vi "colour.vi"(7 "Colour":T2(ring), 8 "error in":errorcluster, 9 "Range":cluster{u32, u32}(slide)={65535, 0} scale=0.0..65535.0, 10 "image":u16[][](array[numeric])) -> (0 "error thru":errorcluster, 2 "picture":picture, 5 "stats":T1={"Histogram"={"X Values"=[5479.58, 5926.74, 6373.9, 6821.06, 7268.22, 7715.38, 8162.54, 8609.7, 9056.86, 9504.02, 9951.18, 10398.34, 10845.5, 11292.66, 11739.82, 12186.98, 12634.14, 13081.3, 13528.46, 13975.62, 14422.78, 14869.94, 15317.1, 15764.26, 16211.42, 16658.58, 17105.74, 17552.9, 18000.06, 18447.22, 18894.38, 19341.54, 19788.7, 20235.86, 20683.02, 21130.18, 21577.34, 22024.5, 22471.66, 22918.82, 23365.98, 23813.14, 24260.3, 24707.46, 25154.62, 25601.78, 26048.94, 26496.1, 26943.26, 27390.42, 27837.58, 28284.74, 28731.9, 29179.06, 29626.22, 30073.38, 30520.54, 30967.7, 31414.86, 31862.02, 32309.18, 32756.34, 33203.5, 33650.66, 34097.82, 34544.98, 34992.14, 35439.3, 35886.46, 36333.62, 36780.78, 37227.94, 37675.1, 38122.26, 38569.42, 39016.58, 39463.74, 39910.9, 40358.06, 40805.22, 41252.38, 41699.54, 42146.7, 42593.86, 43041.02, 43488.18, 43935.34, 44382.5, 44829.66, 45276.82, 45723.98, 46171.14, 46618.3, 47065.46, 47512.62, 47959.78, 48406.94, 48854.1, 49301.26, 49748.42], "Histogram: h(x)"=[2, 4, 12, 22, 46, 28, 40, 61, 53, 89, 50, 76, 48, 43, 66, 54, 64, 43, 68, 121, 142, 240, 196, 324, 218, 283, 392, 283, 484, 412, 686, 750, 950, 1540, 1320, 2011, 1718, 1854, 2735, 2129, 3147, 3035, 5720, 5312, 5580, 7214, 5907, 10090, 10110, 12384, 18538, 16232, 29146, 28690, 37550, 21004, 14573, 14196, 8331, 8677, 4932, 5351, 3336, 2737, 2709, 1284, 1035, 366, 207, 109, 29, 9, 1, 0, 0, 0, 0, 0, 0, 0, 0, 0, 0, 0, 0, 0, 0, 0, 0, 0, 0, 0, 0, 0, 0, 0, 0, 0, 0, 1]}, "max value"=0, "min value"=0})   [LabVIEW 2020]
uses:
  _controls/stats.ctl
  _controls/cluster.range.sgl.ctl
  <vilib>/Analysis/NI_AALBase.lvlib
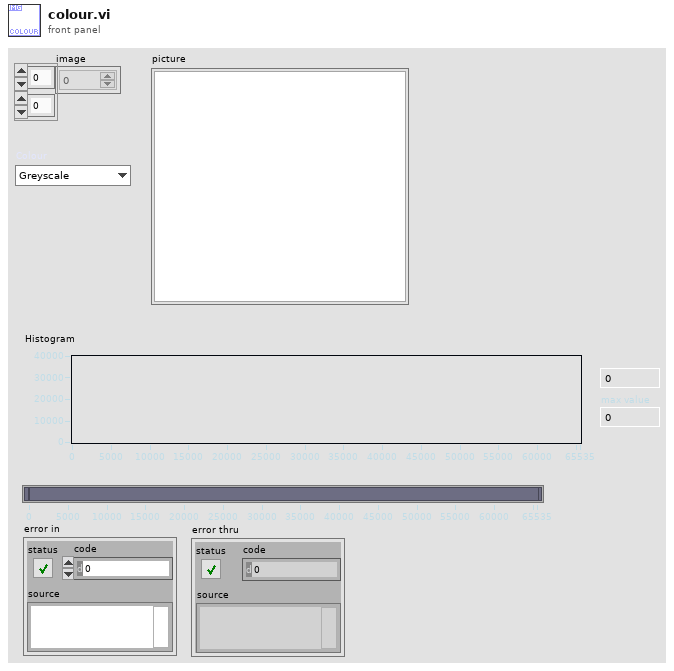
[diagram p1: front panel]
types:
  T1 = typedef "stats.ctl" = cluster{"Histogram":cluster{"X Values":dbl[], "Histogram: h(x)":i32[]}, "max value":u16, "min value":u16}
  T2 = enum16{"Greyscale", "Earth", "Fire", "Rainbow Inverted", "Rainbow", "Red Hot", "Water", "-", "Red", "Orange", "Yellow", "Green", "Cyan", "Blue", "Purple", "Pink"}
  T3 = typedef "cluster.range.sgl.ctl" = cluster{"min":sgl, "max":sgl}
  T4 = cluster{"X Values":dbl[], "Histogram: h(x)":i32[]}
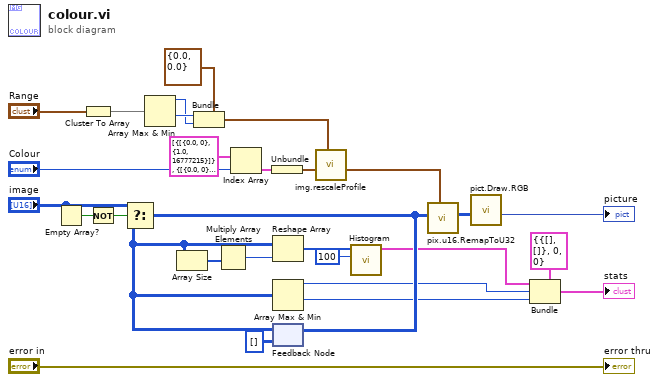
[diagram p0: block diagram]
diagram:
  n1 = Empty Array?(array="image") -> (empty?=w21:bool)
  n2 = Cluster To Array(cluster="Range") -> (array=w1:u32[])
  n3 = Not(x=w21) -> (.not. x?=w20:bool)
  n4 = Array Max & Min(array=w1) -> (max value=w3:u32, min value=w4:u32)  [unwired: 2 out]
  n5 = Bundle(cluster=T3 {"min"=0.0, "max"=0.0} ("range"), "min"=w4, "max"=w3) -> (w2:T3)
  n6 = Index Array(array=cluster{"MarkerValues":cluster{dbl, u32}[]}[] [{"MarkerValues"=[{0.0, 0}, {1.0, 16777215}]}, {"MarkerValues"=[{0.0, 0}, {1.0, 7}, {2.0, 15}, {3.0, 22}, {4.0, 30}, {5.0, 38}, {6.0, 45}, {7.0, 53}, {8.0, 61}, {9.0, 65}, {10.0, 69}, {11.0, 74}, {12.0, 78}, {13.0, 82}, {14.0, 87}, {15.0, 91}, {16.0, 65632}, {17.0, 262244}, {18.0, 458856}, {19.0, 655468}, {20.0, 852081}, {21.0, 1048693}, {22.0, 1245305}, {23.0, 1441917}, {24.0, 1638530}, {25.0, 1835142}, {26.0, 2031754}, {27.0, 2228367}, {28.0, 2424979}, {29.0, 2621591}, {30.0, 2818204}, {31.0, 3014816}, {32.0, 3211429}, {33.0, 3408040}, {34.0, 3604651}, {35.0, 3801263}, {36.0, 3997874}, {37.0, 4194485}, {38.0, 4391097}, {39.0, 4587708}, {40.0, 4784320}, {41.0, 4980931}, {42.0, 5177543}, {43.0, 5374154}, {44.0, 5570766}, {45.0, 5767377}, {46.0, 5963989}, {47.0, 6160600}, {48.0, 6422748}, {49.0, 6619356}, {50.0, 6815965}, {51.0, 7012574}, {52.0, 7209183}, {53.0, 7405792}, {54.0, 7602401}, {55.0, 7799010}, {56.0, 7995619}, {57.0, 8192224}, {58.0, 8388830}, {59.0, 8585436}, {60.0, 8782042}, {61.0, 8978648}, {62.0, 9175254}, {63.0, 9371860}, {64.0, 9568466}, {65.0, 9699534}, {66.0, 9830602}, {67.0, 9961671}, {68.0, 10092739}, {69.0, 10223807}, {70.0, 10354876}, {71.0, 10485944}, {72.0, 10617013}, {73.0, 10682545}, {74.0, 10748077}, {75.0, 10879145}, {76.0, 10944678}, {77.0, 11010210}, {78.0, 11141278}, {79.0, 11206810}, {80.0, 11337879}, {81.0, 11403411}, {82.0, 11468943}, {83.0, 11600012}, {84.0, 11665544}, {85.0, 11731076}, {86.0, 11862145}, {87.0, 11927677}, {88.0, 12058746}, {89.0, 12124278}, {90.0, 12189810}, {91.0, 12320879}, {92.0, 12386411}, {93.0, 12451943}, {94.0, 12583012}, {95.0, 12648544}, {96.0, 12779613}, {97.0, 12845401}, {98.0, 12976981}, {99.0, 13043026}, {100.0, 13174606}, {101.0, 13240394}, {102.0, 13371975}, {103.0, 13438019}, {104.0, 13569600}, {105.0, 13635644}, {106.0, 13701944}, {107.0, 13767989}, {108.0, 13899825}, {109.0, 13966125}, {110.0, 14032170}, {111.0, 14098470}, {112.0, 14230307}, {113.0, 14296351}, {114.0, 14428187}, {115.0, 14494487}, {116.0, 14626324}, {117.0, 14692368}, {118.0, 14824204}, {119.0, 14890504}, {120.0, 15022341}, {121.0, 15088388}, {122.0, 15154691}, {123.0, 15286531}, {124.0, 15352834}, {125.0, 15418881}, {126.0, 15550721}, {127.0, 15617024}, {128.0, 15748864}, {129.0, 15814912}, {130.0, 15946752}, {131.0, 16013056}, {132.0, 16144896}, {133.0, 16210944}, {134.0, 16342784}, {135.0, 16409088}, {136.0, 16540928}, {137.0, 16541440}, {138.0, 16541952}, {139.0, 16608000}, {140.0, 16608512}, {141.0, 16609024}, {142.0, 16675072}, {143.0, 16675584}, {144.0, 16741632}, {145.0, 16742144}, {146.0, 16742656}, {147.0, 16743168}, {148.0, 16743680}, {149.0, 16744192}, {150.0, 16744704}, {151.0, 16745216}, {152.0, 16745728}, {153.0, 16745984}, {154.0, 16746496}, {155.0, 16747008}, {156.0, 16747520}, {157.0, 16747776}, {158.0, 16748288}, {159.0, 16748800}, {160.0, 16749312}, {161.0, 16749568}, {162.0, 16750080}, {163.0, 16750592}, {164.0, 16751104}, {165.0, 16751360}, {166.0, 16751872}, {167.0, 16752384}, {168.0, 16752896}, {169.0, 16753152}, {170.0, 16753664}, {171.0, 16754176}, {172.0, 16754688}, {173.0, 16754944}, {174.0, 16755456}, {175.0, 16755968}, {176.0, 16756480}, {177.0, 16756736}, {178.0, 16757248}, {179.0, 16757760}, {180.0, 16758272}, {181.0, 16758784}, {182.0, 16759296}, {183.0, 16759808}, {184.0, 16760320}, {185.0, 16760576}, {186.0, 16761088}, {187.0, 16761600}, {188.0, 16762112}, {189.0, 16762624}, {190.0, 16763136}, {191.0, 16763648}, {192.0, 16764160}, {193.0, 16764416}, {194.0, 16764928}, {195.0, 16765440}, {196.0, 16765952}, {197.0, 16766208}, {198.0, 16766720}, {199.0, 16767232}, {200.0, 16767744}, {201.0, 16768000}, {202.0, 16768512}, {203.0, 16769024}, {204.0, 16769536}, {205.0, 16770048}, {206.0, 16770560}, {207.0, 16771072}, {208.0, 16771584}, {209.0, 16771844}, {210.0, 16772360}, {211.0, 16772877}, {212.0, 16773393}, {213.0, 16773653}, {214.0, 16774170}, {215.0, 16774686}, {216.0, 16775203}, {217.0, 16775210}, {218.0, 16775474}, {219.0, 16775738}, {220.0, 16776002}, {221.0, 16776266}, {222.0, 16776530}, {223.0, 16776794}, {224.0, 16777058}, {225.0, 16777065}, {226.0, 16777073}, {227.0, 16777081}, {228.0, 16777089}, {229.0, 16777096}, {230.0, 16777104}, {231.0, 16777112}, {232.0, 16777120}, {233.0, 16777127}, {234.0, 16777135}, {235.0, 16777143}, {236.0, 16777151}, {237.0, 16777159}, {238.0, 16777167}, {239.0, 16777175}, {240.0, 16777183}, {241.0, 16777187}, {242.0, 16777191}, {243.0, 16777195}, {244.0, 16777199}, {245.0, 16777203}, {246.0, 16777207}, {247.0, 16777211}, {248.0, 16777215}, {249.0, 16777215}, {250.0, 16777215}, {251.0, 16777215}, {252.0, 16777215}, {253.0, 16777215}, {254.0, 16777215}, {255.0, 16777215}]}, {"MarkerValues"=[{0.0, 0}, {21845.0, 16744277}, {43690.0, 16777130}, {65535.0, 16777215}]}, {"MarkerValues"=[{6.0, 63}, {5.0, 255}, {4.0, 65535}, {3.0, 65280}, {2.0, 16776960}, {1.0, 16711680}, {0.0, 8323072}]}, {"MarkerValues"=[{0.0, 0}, {1.0, 255}, {2.0, 65535}, {3.0, 65280}, {4.0, 16776960}, {5.0, 16711680}, {6.0, 8323072}]}, {"MarkerValues"=[{0.0, 0}, {1.0, 0}, {2.0, 0}, {3.0, 0}, {4.0, 65793}, {5.0, 65793}, {6.0, 65793}, {7.0, 65793}, {8.0, 65793}, {9.0, 262144}, {10.0, 458752}, {11.0, 655360}, {12.0, 851968}, {13.0, 1048576}, {14.0, 1310720}, {15.0, 1507328}, {16.0, 1769472}, {17.0, 1966080}, {18.0, 2162688}, {19.0, 2359296}, {20.0, 2555904}, {21.0, 2752512}, {22.0, 2949120}, {23.0, 3145728}, {24.0, 3407872}, {25.0, 3604480}, {26.0, 3801088}, {27.0, 3997696}, {28.0, 4259840}, {29.0, 4456448}, {30.0, 4653056}, {31.0, 4849664}, {32.0, 5111808}, {33.0, 5308416}, {34.0, 5505024}, {35.0, 5701632}, {36.0, 5898240}, {37.0, 6094848}, {38.0, 6291456}, {39.0, 6488064}, {40.0, 6750208}, {41.0, 6946816}, {42.0, 7208960}, {43.0, 7405568}, {44.0, 7667712}, {45.0, 7864320}, {46.0, 8060928}, {47.0, 8257536}, {48.0, 8519680}, {49.0, 8716288}, {50.0, 8912896}, {51.0, 9109504}, {52.0, 9306112}, {53.0, 9502720}, {54.0, 9699328}, {55.0, 9895936}, {56.0, 10158080}, {57.0, 10354688}, {58.0, 10551296}, {59.0, 10747904}, {60.0, 11010048}, {61.0, 11206656}, {62.0, 11403264}, {63.0, 11599872}, {64.0, 11862016}, {65.0, 12058624}, {66.0, 12255232}, {67.0, 12451840}, {68.0, 12648448}, {69.0, 12845056}, {70.0, 13107200}, {71.0, 13303808}, {72.0, 13565952}, {73.0, 13762560}, {74.0, 13959168}, {75.0, 14155776}, {76.0, 14417920}, {77.0, 14614528}, {78.0, 14811136}, {79.0, 15007744}, {80.0, 15269888}, {81.0, 15466496}, {82.0, 15663104}, {83.0, 15859712}, {84.0, 16056320}, {85.0, 16187392}, {86.0, 16384256}, {87.0, 16515584}, {88.0, 16712448}, {89.0, 16713216}, {90.0, 16713984}, {91.0, 16714752}, {92.0, 16715776}, {93.0, 16716544}, {94.0, 16717312}, {95.0, 16718080}, {96.0, 16719104}, {97.0, 16719872}, {98.0, 16720640}, {99.0, 16721408}, {100.0, 16722432}, {101.0, 16723200}, {102.0, 16723968}, {103.0, 16724736}, {104.0, 16725760}, {105.0, 16726528}, {106.0, 16727296}, {107.0, 16728064}, {108.0, 16729088}, {109.0, 16729856}, {110.0, 16730624}, {111.0, 16731392}, {112.0, 16732416}, {113.0, 16733184}, {114.0, 16733952}, {115.0, 16734720}, {116.0, 16735744}, {117.0, 16736512}, {118.0, 16737280}, {119.0, 16738048}, {120.0, 16738816}, {121.0, 16739584}, {122.0, 16740352}, {123.0, 16741120}, {124.0, 16742144}, {125.0, 16742912}, {126.0, 16743936}, {127.0, 16744704}, {128.0, 16745728}, {129.0, 16746496}, {130.0, 16747264}, {131.0, 16748032}, {132.0, 16748800}, {133.0, 16749568}, {134.0, 16750336}, {135.0, 16751104}, {136.0, 16752128}, {137.0, 16752896}, {138.0, 16753664}, {139.0, 16754432}, {140.0, 16755456}, {141.0, 16756224}, {142.0, 16756992}, {143.0, 16757760}, {144.0, 16758784}, {145.0, 16759552}, {146.0, 16760320}, {147.0, 16761088}, {148.0, 16762112}, {149.0, 16762880}, {150.0, 16763648}, {151.0, 16764416}, {152.0, 16765184}, {153.0, 16765952}, {154.0, 16766976}, {155.0, 16767744}, {156.0, 16768768}, {157.0, 16769536}, {158.0, 16770304}, {159.0, 16771072}, {160.0, 16772096}, {161.0, 16772864}, {162.0, 16773632}, {163.0, 16774400}, {164.0, 16775424}, {165.0, 16775681}, {166.0, 16776195}, {167.0, 16776452}, {168.0, 16776966}, {169.0, 16776969}, {170.0, 16776972}, {171.0, 16776975}, {172.0, 16776979}, {173.0, 16776982}, {174.0, 16776985}, {175.0, 16776988}, {176.0, 16776992}, {177.0, 16776995}, {178.0, 16776998}, {179.0, 16777001}, {180.0, 16777005}, {181.0, 16777008}, {182.0, 16777011}, {183.0, 16777014}, {184.0, 16777018}, {185.0, 16777021}, {186.0, 16777024}, {187.0, 16777027}, {188.0, 16777031}, {189.0, 16777034}, {190.0, 16777037}, {191.0, 16777040}, {192.0, 16777044}, {193.0, 16777047}, {194.0, 16777050}, {195.0, 16777053}, {196.0, 16777057}, {197.0, 16777060}, {198.0, 16777063}, {199.0, 16777066}, {200.0, 16777070}, {201.0, 16777073}, {202.0, 16777076}, {203.0, 16777079}, {204.0, 16777082}, {205.0, 16777085}, {206.0, 16777088}, {207.0, 16777091}, {208.0, 16777095}, {209.0, 16777098}, {210.0, 16777102}, {211.0, 16777105}, {212.0, 16777109}, {213.0, 16777112}, {214.0, 16777115}, {215.0, 16777118}, {216.0, 16777121}, {217.0, 16777124}, {218.0, 16777127}, {219.0, 16777130}, {220.0, 16777134}, {221.0, 16777137}, {222.0, 16777140}, {223.0, 16777143}, {224.0, 16777147}, {225.0, 16777150}, {226.0, 16777153}, {227.0, 16777156}, {228.0, 16777160}, {229.0, 16777163}, {230.0, 16777166}, {231.0, 16777169}, {232.0, 16777173}, {233.0, 16777176}, {234.0, 16777179}, {235.0, 16777182}, {236.0, 16777185}, {237.0, 16777188}, {238.0, 16777192}, {239.0, 16777195}, {240.0, 16777199}, {241.0, 16777202}, {242.0, 16777205}, {243.0, 16777208}, {244.0, 16777212}, {245.0, 16777212}, {246.0, 16777213}, {247.0, 16777214}, {248.0, 16777215}, {249.0, 16777215}, {250.0, 16777215}, {251.0, 16777215}, {252.0, 16777215}, {253.0, 16777215}, {254.0, 16777215}, {255.0, 16777215}]}, {"MarkerValues"=[{0.0, 0}, {1.0, 255}, {2.0, 16777215}]}, {"MarkerValues"=[]}, {"MarkerValues"=[{0.0, 0}, {1.0, 16711680}]}, {"MarkerValues"=[{0.0, 0}, {1.0, 16744448}]}, {"MarkerValues"=[{0.0, 0}, {1.0, 16776960}]}, {"MarkerValues"=[{0.0, 0}, {1.0, 65280}]}, {"MarkerValues"=[{0.0, 0}, {1.0, 65535}]}, {"MarkerValues"=[{0.0, 0}, {1.0, 33023}]}, {"MarkerValues"=[{0.0, 0}, {1.0, 12583167}]}, {"MarkerValues"=[{0.0, 0}, {1.0, 16711872}]}] ("profiles"), index="Colour") -> (element=w24:cluster{"MarkerValues":cluster{dbl, u32}[]})
  n7 = Unbundle(w24) -> ("MarkerValues"=w25:cluster{dbl, u32}[])
  n8 = feedback #1(u16[][] [] ("img.24bit")) -> (w13:u16[][])
  n9 = Select(t="image", s=w20, f=w13) -> (s? t:f=w12:u16[][])
  n10 = Array Size(array=w13) -> (size(s)=w15:i32[])
  n11 = Multiply Array Elements(1:w15) -> (0:w14:i32)
  n12 = Reshape Array(w13, w14) -> (w17:u16[])
  n13 = Array Max & Min(array=w13) -> (max value=w10:u16, min value=w11:u16)  [unwired: 2 out]
  n14 = feedback-in #1(w12) -> ()
  n15 = call "img.rescaleProfile.vi"("range"=w2, "MarkerVals in (greyscale)"=w25) -> ("MarkerVals out"=w23:cluster{dbl, u32}[])  [unwired: 8 in, 1 out]
  n16 = call <vilib>:"Histogram.vi"("intervals"=100, "X"=w17) -> ("Histogram Graph"=w8:T4)  [unwired: 6 in, 3 out]
  n17 = call "pix.u16.RemapToU32.vi"("ZScale.MarkerValues"=w23, "img.u16"=w12) -> ("img.24bit"=w27:u32[][])  [unwired: 7 in]
  n18 = call "pict.Draw.RGB.vi"("RGB pixmap"=w27) -> ("picture"=→"picture":picture)  [unwired: 10 in]
  n19 = Bundle(cluster=T1 {"Histogram"={"X Values"=[], "Histogram: h(x)"=[]}, "max value"=0, "min value"=0} ("stats"), "Histogram"=w8, "max value"=w10, "min value"=w11) -> (→"stats":T1)
  "error thru" <- "error in"
